vi "Soft Smooth.vi"(1 "current y":dbl[](array[numeric]), 2 "# of Smooths":i32) -> (0 "new y":dbl[](array[numeric]))   [LabVIEW 2012]
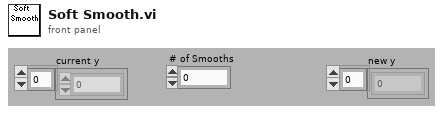
[diagram p1: front panel]
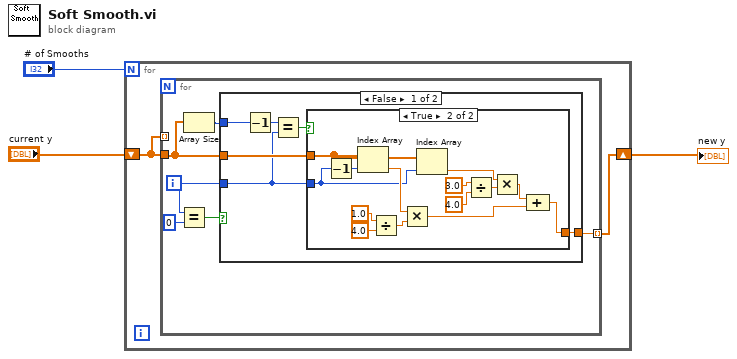
[diagram p0: block diagram]
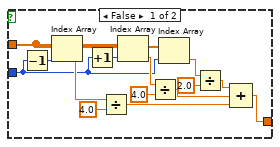
[diagram p2: hidden frame]
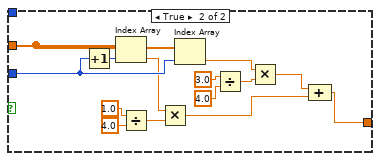
[diagram p3: hidden frame]
diagram:
  n1 = for {
    N: "# of Smooths" -> [_]
    shift-right: [w5] -> w3
    shift-left: "current y" -> [w4]
    n2 = for {
      tunnel: w4 -> [w7]
      tunnel: [w11] -> w5 mode=indexing
      tunnel: w4 -> [_] mode=indexing
      i -> [w9]
      n3 = Equal?(x=w9, y=0) -> (x = y?=w10:bool)
      n4 = Array Size(array=w7) -> (size(s)=w6:i32)
      n5 = case shown="False" w10 {
        tunnel: w7 -> [w16 w56]
        tunnel: [w17 w55] -> w11
        tunnel: w9 -> [w12 w54]
        tunnel: w6 -> [w14 _]
        frame False {
          n6 = Decrement(x=w14) -> (x-1=w13:i32)
          n7 = Equal?(x=w13, y=w12) -> (x = y?=w15:bool)
          n8 = case shown="True" w15 {
            tunnel: w16 -> [w29 w36]
            tunnel: [w24 w34] -> w17
            tunnel: w12 -> [w18 w35]
            frame False {
              n9 = Decrement(x=w18) -> (x-1=w31:i32)
              n10 = Index Array(array=w29, index=w31) -> (element=w27:dbl)
              n11 = Increment(x=w18) -> (x+1=w30:i32)
              n12 = Divide(x=w27, y=4.0) -> (x/y=w23:dbl)
              n13 = Index Array(array=w29, index=w30) -> (element=w28:dbl)
              n14 = Divide(x=w28, y=4.0) -> (x/y=w22:dbl)
              n15 = Index Array(array=w29, index=w18) -> (element=w20:dbl)
              n16 = Divide(x=w20, y=2.0) -> (x/y=w21:dbl)
              n17 = Compound Arithmetic op=ADD(w21, w22, w23) -> (w24:dbl)
            }
            frame True {
              n18 = Decrement(x=w35) -> (x-1=w45:i32)
              n19 = Index Array(array=w36, index=w45) -> (element=w40:dbl)
              n20 = Divide(x=1.0 ("y"), y=4.0) -> (x/y=w33:dbl)
              n21 = Multiply(x=w40, y=w33) -> (x*y=w41:dbl)
              n22 = Index Array(array=w36, index=w35) -> (element=w37:dbl)
              n23 = Divide(x=3.0 ("y"), y=4.0) -> (x/y=w32:dbl)
              n24 = Multiply(x=w37, y=w32) -> (x*y=w38:dbl)
              n25 = Compound Arithmetic op=ADD(w38, w41) -> (w34:dbl)
            }
          }
        }
        frame True {
          n26 = Increment(x=w54) -> (x+1=w59:i32)
          n27 = Index Array(array=w56, index=w59) -> (element=w51:dbl)
          n28 = Divide(x=1.0 ("y"), y=4.0) -> (x/y=w46:dbl)
          n29 = Multiply(x=w51, y=w46) -> (x*y=w52:dbl)
          n30 = Index Array(array=w56, index=w54) -> (element=w48:dbl)
          n31 = Divide(x=3.0 ("y"), y=4.0) -> (x/y=w47:dbl)
          n32 = Multiply(x=w48, y=w47) -> (x*y=w49:dbl)
          n33 = Compound Arithmetic op=ADD(w49, w52) -> (w55:dbl)
        }
      }
    }
  }
  "new y" <- w3
